vi "test - float format.vi"(8 "error in (no error)":errorcluster, 11 "TestCase in":refnum<class "testcase-Supported-Datatype.lvclass">) -> (0 "error out":errorcluster, 3 "TestCase out":refnum<class "testcase-Supported-Datatype.lvclass">)   [LabVIEW 2017, in "testcase-Supported-Datatype.lvclass"]
uses:
  testcase-Supported-Datatype.lvclass
  2a298ae6-dd3b-42b5-90b2-6aeb4f0b9897.vi
  addons/API-String-Arugments-Support/_Support/Data To API String Arguments.vi
  <vilib>/addons/_JKI Toolkits/VI Tester/TestCase.llb/TestCase.lvclass
  addons/API-String-Arugments-Support/API String Arguments Support.lvlib
  C:/Program Files (x86)/National Instruments/LabVIEW 2017/vi.lib/addons/_JKI Toolkits/VI Tester/TestCase.llb/TestCase.lvclass
panel:
  out "Array":string[](array[string])
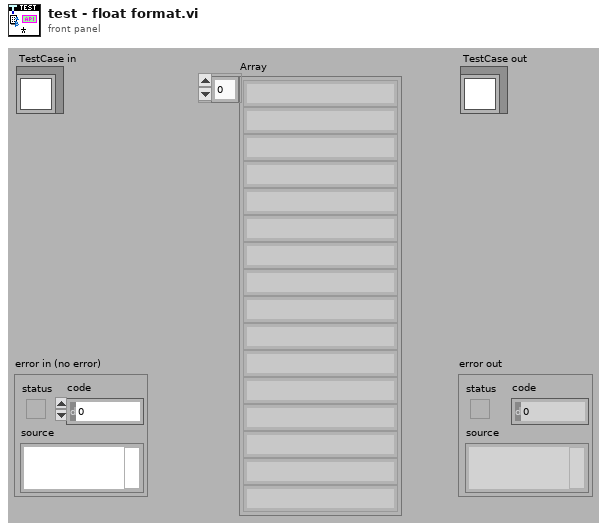
[diagram p1: front panel]
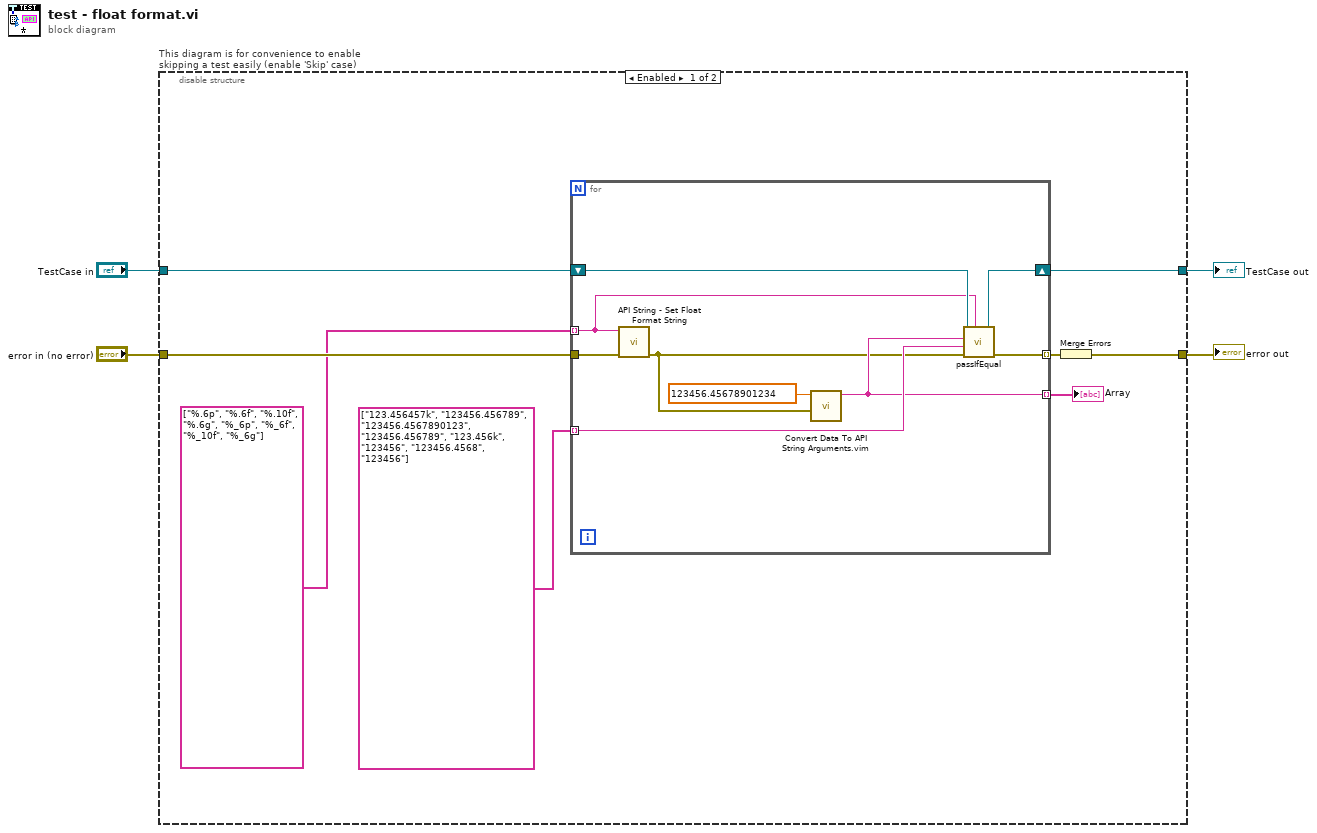
[diagram p0: block diagram]
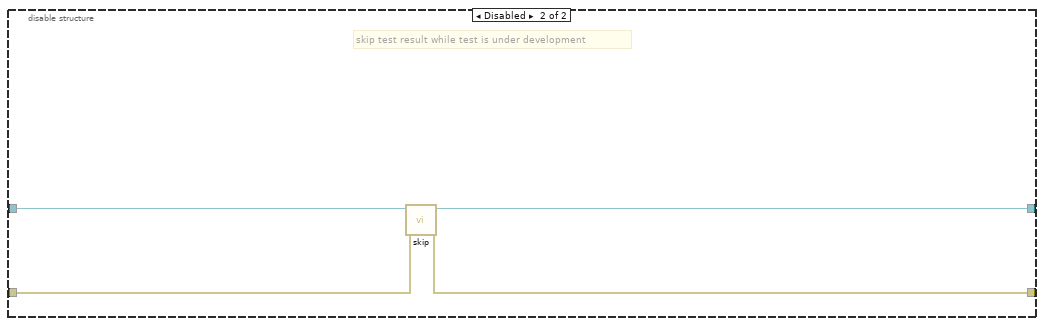
[diagram p2: hidden frame]
diagram:
  n1 = disable-structure "This diagram is for convenience to enable skipping a test easily (enable 'Skip' case)" shown="Enabled" {
    disable-tunnel: "TestCase in" -> [w12 w25]
    disable-tunnel: [w10 w23] -> w1
    disable-tunnel: [w5 w24] -> w3
    disable-tunnel: "error in (no error)" -> [w11 w22]
    frame Enabled {
      n2 = for {
        shift-right: [w19] -> w10
        shift-left: w12 -> [w21]
        tunnel: string[] ["%.6p", "%.6f", "%.10f", "%.6g", "%_6p", "%_6f", "%_10f", "%_6g"] ("Float Format String Setting") -> [w14] mode=indexing
        tunnel: string[] ["123.456457k", "123456.456789", "123456.4567890123", "123456.456789", "123.456k", "123456", "123456.4568", "123456"] ("Float Format String Setting") -> [w16] mode=indexing
        tunnel: [w15] -> w6 mode=indexing
        tunnel: w11 -> [w20]
        tunnel: [w18] -> w9 mode=indexing
        n3 = call "API String - Set Float Format String.vi"("Error in"=w20, "Float Format String Setting"=w14) -> ("Error out"=w13:errorcluster)  [unwired: 8 in, 1 out]
        n4 = call "Convert Data To API String Arguments.vim"("error in (no error)"=w13, "Data"=123456.45678901234) -> ("API String"=w15:string)  [unwired: 6 in, 1 out]
        n5 = call-dynamic "passIfEqual.vi"("custom report message (\"\")"=w14, "error in (no error)"=w13, "y"=w16, "x"=w15, "TestCase in"=w21) -> ("error out"=w18:errorcluster, "TestCase out"=w19:refnum<class "testcase-Supported-Datatype.lvclass">)  [unwired: 5 in]
      }
      "Array" <- w6
      n6 = Merge Errors(w9) -> (w5:errorcluster)
    }
    frame Disabled {
      # "skip test result while test is under development"
      n7 = call <vilib>:"skip.vi"("error in (no error)"=w22, "TestCase in"=w25) -> ("error out"=w24:errorcluster, "TestCase out"=w23:refnum<class "testcase-Supported-Datatype.lvclass">)  [unwired: 8 in]
    }
  }
  "error out" <- w3
  "TestCase out" <- w1
